vi "replace_boolean_with_on_off.vi"(8 "error in (no error)":errorcluster, 11 "String In":string) -> (0 "error out":errorcluster, 3 "String Out":string)   [LabVIEW 2018]
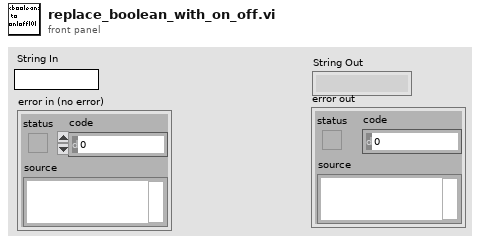
[diagram p1: front panel]
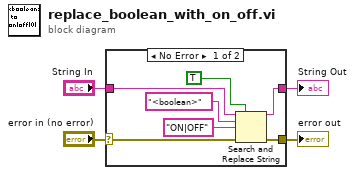
[diagram p0: block diagram]
diagram:
  n1 = case shown="No Error" "error in (no error)" {
    selector: "error in (no error)" -> [w7 w12]
    tunnel: "String In" -> [w11 w13]
    tunnel: [w8 w13] -> w3
    tunnel: [w6 w12] -> w1
    frame No Error {
      n2 = Search and Replace String(replace all?=TRUE ("replace all? (F)"), input string=w11, search string="<boolean>", replace string="ON|OFF" ("replace string (\"\")"), error in=w7) -> (result string=w8:string, error out=w6:errorcluster)  [unwired: 5 out]
    }
    frame Error {
    }
  }
  "String Out" <- w3
  "error out" <- w1
